vi "ZAlign_End.vi"(0 "Panel in":refnum<vi>, 5 "VI in":refnum<vi>, 11 "error in (no error)":errorcluster) -> (15 "error out":errorcluster)   [LabVIEW 2014, in "ZAlign.lvlib"]
doc: "ZAlign.lvlib:ZAlign_End.vi\n----------------------------------------------\nEnde des Quickdrops.\n\nInputs:\n---------------------\n- Panel in : Refnum; \n- VI in : Refnum; \n- error in (no error) : Cluster; \n\nOutputs:\n---------------------\n- error out : Cluster; \n\n----------------------------------------------\n26.03.2015 jcm\nZühlke Engineering AG\nCH-8952 Schlieren\nwww.zuehlke.com"
uses:
  ZAlign.lvlib
panel:
  # "Connector Pane"
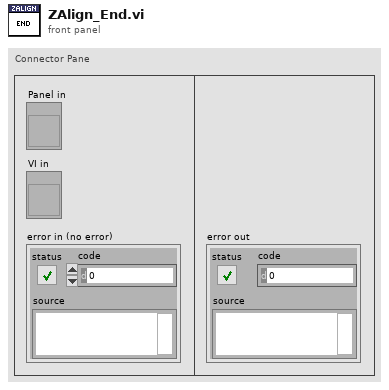
[diagram p1: front panel]
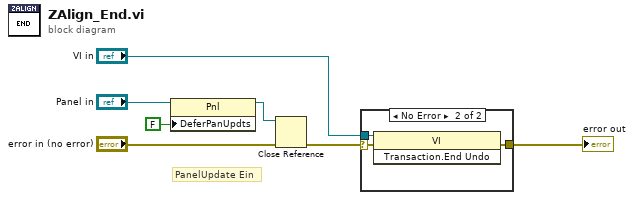
[diagram p0: block diagram]
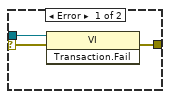
[diagram p2: hidden frame]
diagram:
  # "PanelUpdate Ein"
  n1 = property class="Pnl"(reference="Panel in", "DeferPanUpdts"=FALSE ("Defer Panel Updates")) -> (reference out=w7:refnum<vi>)  [unwired: 1 in, 1 out]
  n2 = Close Reference(reference=w7, error in (no error)="error in (no error)") -> (error out=w5:errorcluster)
  n3 = case shown="No Error" w5 {
    selector: w5 -> [w8 w11]
    tunnel: "VI in" -> [w9 w12]
    tunnel: [w10 w13] -> w1
    frame Error {
      n4 = invoke class="VI" method="Transaction.Fail"(reference=w9, error in=w8) -> (error out=w10:errorcluster)  [unwired: 1 in, 2 out]
    }
    frame No Error {
      n5 = invoke class="VI" method="Transaction.End Undo"(reference=w12, error in=w11) -> (error out=w13:errorcluster)  [unwired: 1 in, 2 out]
    }
  }
  "error out" <- w1
